vi "测量数据区.vi"(11 "数组":u16[](array[numeric]) format="%04xH") -> (3 "测量数据区":T1 {"单位" items=["ug/L", "mg/L", "ppm", "mg/m3", "cm", "ppb", "ug/m3", "%", "nmol/mol", "umol/mol", "MPN/L", "MPN/100ml", "ng/m3", "NTU", "无量纲", "ms/cm", "us/cm", "℃", "mV", "万个/L"]})   [LabVIEW 2016, in "斯坦道CODcr.lvlib"]
panel:
  # "共占用105 WORD"
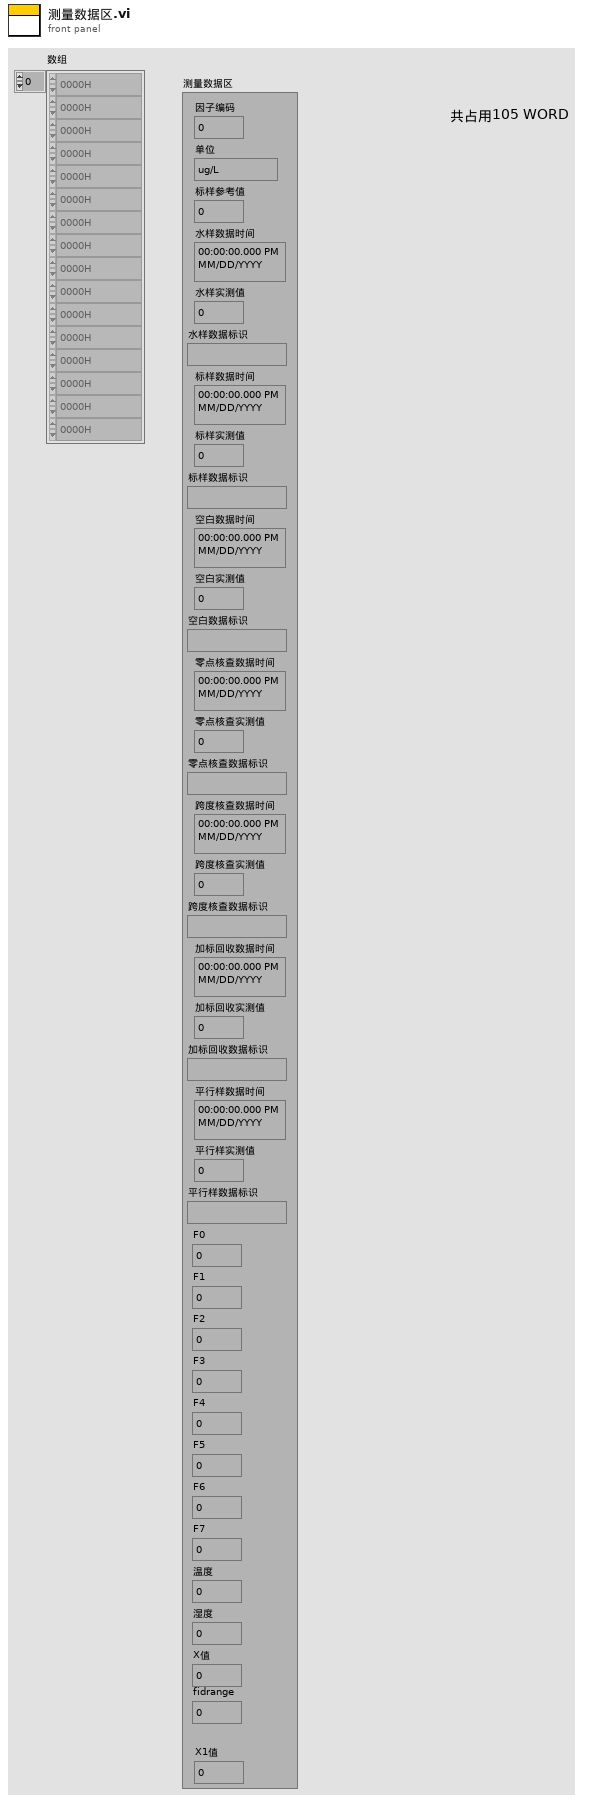
[diagram p1: front panel]
types:
  T1 = cluster{"因子编码":u32, "单位":u16, "标样参考值":sgl, "水样数据时间":timestamp, "水样实测值":sgl, "水样数据标识":string, "标样数据时间":timestamp, "标样实测值":sgl, "标样数据标识":string, "空白数据时间":timestamp, "空白实测值":sgl, "空白数据标识":string, "零点核查数据时间":timestamp, "零点核查实测值":sgl, "零点核查数据标识":string, "跨度核查数据时间":timestamp, "跨度核查实测值":sgl, "跨度核查数据标识":string, "加标回收数据时间":timestamp, "加标回收实测值":sgl, "加标回收数据标识":string, "平行样数据时间":timestamp, "平行样实测值":sgl, "平行样数据标识":string, "F0":sgl, "F1":sgl, "F2":sgl, "F3":sgl, "F4":sgl, "F5":sgl, "F6":sgl, "F7":sgl, "温度":sgl, "湿度":sgl, "X值":sgl, "fidrange":u16, "X1值":sgl}
  T2 = cluster{"DWORD":i32, "WORD":u16, "FLOAT":sgl, "time stamp":timestamp, "数值":sgl, "string":string, "time stamp":timestamp, "数值":sgl, "string":string, "time stamp":timestamp, "数值":sgl, "string":string, "time stamp":timestamp, "数值":sgl, "string":string, "time stamp":timestamp, "数值":sgl, "string":string, "time stamp":timestamp, "数值":sgl, "string":string, "time stamp":timestamp, "数值":sgl, "string":string, "FLOAT":sgl, "FLOAT":sgl, "FLOAT":sgl, "FLOAT":sgl, "FLOAT":sgl, "FLOAT":sgl, "FLOAT":sgl, "FLOAT":sgl, "FLOAT":sgl, "FLOAT":sgl, "FLOAT":sgl, "数值":u16, "FLOAT":sgl}
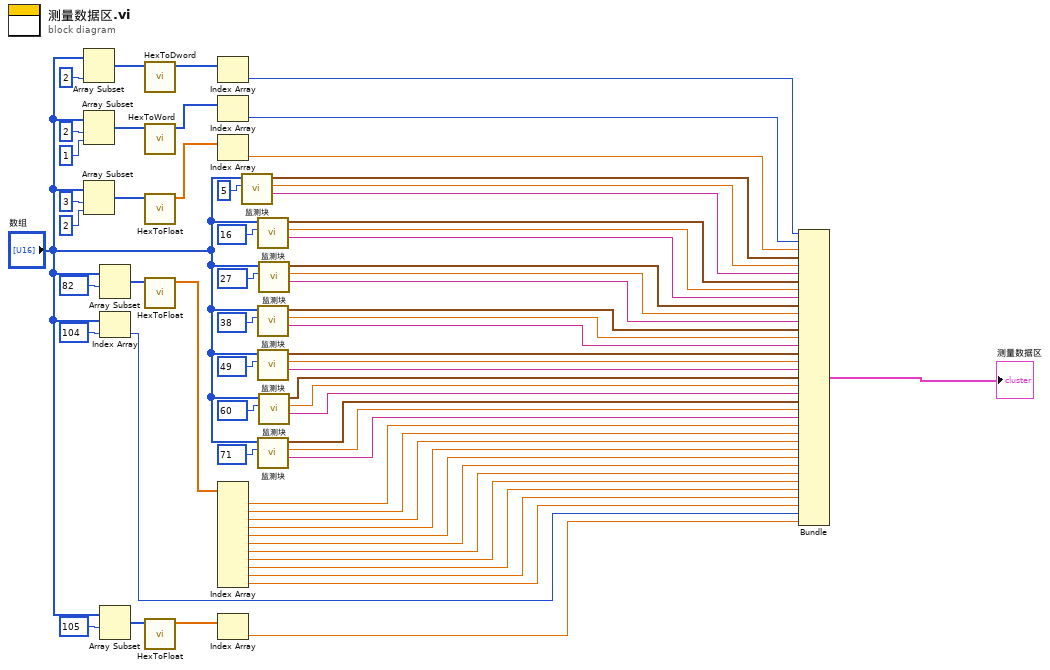
[diagram p0: block diagram]
diagram:
  n1 = Array Subset(array="数组", length=2 ("长度")) -> (w64:u16[])  [unwired: 1 in]
  n2 = Array Subset(array="数组", index=2 ("索引"), length=1 ("长度")) -> (w59:u16[])
  n3 = Array Subset(array="数组", index=3 ("索引"), length=2 ("长度")) -> (w54:u16[])
  n4 = Array Subset(array="数组", index=82 ("索引")) -> (w20:u16[])  [unwired: 1 in]
  n5 = Index Array(array="数组", index=104 ("索引")) -> (element=w6:u16)
  n6 = Array Subset(array="数组", index=105 ("索引")) -> (w3:u16[])  [unwired: 1 in]
  n7 = call "HexToDword.vi"("数组"=w64) -> ("DWORD"=w62:i32[])  [unwired: 10 in]
  n8 = call "HexToWord.vi"("数组"=w59) -> ("WORD"=w58:u16[])  [unwired: 10 in]
  n9 = call "HexToFloat.vi"("数组"=w54) -> ("FLOAT"=w53:sgl[])  [unwired: 10 in]
  n10 = call "HexToFloat.vi"("数组"=w20) -> ("FLOAT"=w19:sgl[])  [unwired: 10 in]
  n11 = call "HexToFloat.vi"("数组"=w3) -> ("FLOAT"=w2:sgl[])  [unwired: 10 in]
  n12 = Index Array(array=w62) -> (element=w23:i32)  [unwired: 1 in]
  n13 = Index Array(array=w58) -> (element=w57:u16)  [unwired: 1 in]
  n14 = Index Array(array=w53) -> (element=w52:sgl)  [unwired: 1 in]
  n15 = Index Array(array=w19) -> (element #1=w18:sgl, element #2=w17:sgl, element #3=w16:sgl, element #4=w15:sgl, element #5=w14:sgl, element #6=w13:sgl, element #7=w12:sgl, element #8=w11:sgl, element #9=w10:sgl, element #10=w9:sgl, element #11=w8:sgl)  [unwired: 11 in]
  n16 = Index Array(array=w2) -> (element=w1:sgl)  [unwired: 1 in]
  n17 = call "监测块.vi"("索引"=5, "数组"="数组") -> ("string"=w49:string, "数值"=w50:sgl, "time stamp"=w51:timestamp)  [unwired: 7 in]
  n18 = call "监测块.vi"("索引"=16, "数组"="数组") -> ("string"=w44:string, "数值"=w45:sgl, "time stamp"=w46:timestamp)  [unwired: 7 in]
  n19 = call "监测块.vi"("索引"=38, "数组"="数组") -> ("string"=w36:string, "数值"=w37:sgl, "time stamp"=w38:timestamp)  [unwired: 7 in]
  n20 = call "监测块.vi"("索引"=49, "数组"="数组") -> ("string"=w32:string, "数值"=w33:sgl, "time stamp"=w34:timestamp)  [unwired: 7 in]
  n21 = call "监测块.vi"("索引"=71, "数组"="数组") -> ("string"=w24:string, "数值"=w25:sgl, "time stamp"=w26:timestamp)  [unwired: 7 in]
  n22 = call "监测块.vi"("索引"=27, "数组"="数组") -> ("string"=w40:string, "数值"=w41:sgl, "time stamp"=w42:timestamp)  [unwired: 7 in]
  n23 = call "监测块.vi"("索引"=60, "数组"="数组") -> ("string"=w28:string, "数值"=w29:sgl, "time stamp"=w30:timestamp)  [unwired: 7 in]
  n24 = Bundle("DWORD"=w23, "WORD"=w57, "FLOAT"=w52, "time stamp"=w51, "数值"=w50, "string"=w49, "time stamp"=w46, "数值"=w45, "string"=w44, "time stamp"=w42, "数值"=w41, "string"=w40, "time stamp"=w38, "数值"=w37, "string"=w36, "time stamp"=w34, "数值"=w33, "string"=w32, "time stamp"=w30, "数值"=w29, "string"=w28, "time stamp"=w26, "数值"=w25, "string"=w24, "FLOAT"=w18, "FLOAT"=w17, "FLOAT"=w16, "FLOAT"=w15, "FLOAT"=w14, "FLOAT"=w13, "FLOAT"=w12, "FLOAT"=w11, "FLOAT"=w10, "FLOAT"=w9, "FLOAT"=w8, "数值"=w6, "FLOAT"=w1) -> (→"测量数据区":T2)  [unwired: 1 in]
